vi "Condicion1.vi"(0 "KickToSkill in":refnum<class "KickToSkill.lvclass">, 1 "R-B norm":dbl, 2 "R-T":dbl[](array[numeric]), 3 "error in (no error)":errorcluster, 4 "Raio":dbl) -> (5 "Boolean":bool)   [LabVIEW 2021, in "KickToSkill.lvclass"]
uses:
  KickToSkill.lvclass
  <vilib>/Analysis/coordinate.llb/2D Cartesian Coordinate Rotation (Scalar).vi
  <vilib>/Analysis/NI_AALPro.lvlib
panel:
  in  "R-B":dbl[](array[numeric])
  out "KickToSkill out":refnum<class "KickToSkill.lvclass">
  out "error out":errorcluster
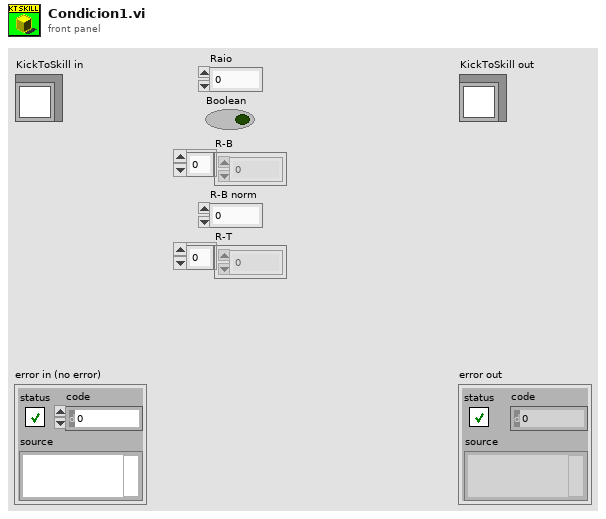
[diagram p1: front panel]
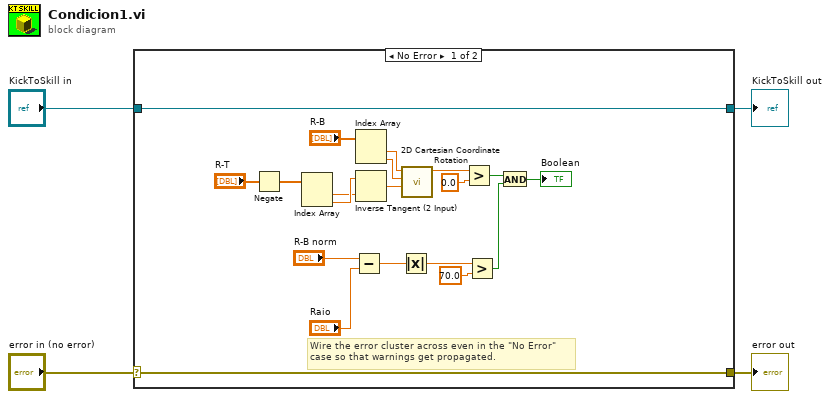
[diagram p0: block diagram]
diagram:
  n1 = case shown="No Error" "error in (no error)" {
    selector: "error in (no error)" -> [w23 w26]
    tunnel: [w23 w26] -> w3
    tunnel: [w24 w25] -> w1
    tunnel: "KickToSkill in" -> [w24 w25]
    frame No Error {
      # "Wire the error cluster across even in the \"No Error\"\ncase so that warnings get propagated."
      n2 = Negate(x="R-T") -> (-x=w9:dbl[])
      n3 = Index Array(array=w9) -> (element #1=w6:dbl, element #2=w7:dbl)  [unwired: 2 in]
      n4 = Subtract(x="R-B norm", y="Raio") -> (x-y=w17:dbl)
      n5 = Index Array(array="R-B") -> (element #1=w11:dbl, element #2=w12:dbl)  [unwired: 2 in]
      n6 = Inverse Tangent (2 Input)(1:w6, 2:w7) -> (0:w5:dbl)
      n7 = Absolute Value(x=w17) -> (abs(x)=w18:dbl)
      n8 = call-poly <vilib>:"2D Cartesian Coordinate Rotation.vi"("theta"=w5, "y"=w12, "x"=w11) -> ("x out"=w13:dbl)  [unwired: 6 in, 2 out]
      n9 = Greater?(x=w13, y=0.0) -> (0:w20:bool)
      n10 = Greater?(x=w18, y=70.0) -> (0:w21:bool)
      n11 = And(x=w20, y=w21) -> (x .and. y?=→"Boolean":bool)
    }
    frame Error {
    }
  }
  "error out" <- w3
  "KickToSkill out" <- w1
